vi "recon_zern_fileIO_MATLAB_v2.vi"(0 "Number of Phase":u32=2, 1 "Number for average":u32=2, 3 "Crop Size of image":u32=384, 4 "Background Value":u32=290, 5 "Zernike Order":u32=15, 7 "error in (no error)":errorcluster, 8 "Use GPU":bool=TRUE, 9 "Iteration Number":u32=10, 10 "idxType":enum16{"Wyant", "ANSI"}(ring), 12 "File Name":string="beads_1", 13 "Gamma Value":dbl=1e-06, 14 "Path In":path=path "D:/Data", 15 "Show Input":bool, 16 "Path Out":path=path "D:/Data", 17 "Show Recon":bool=TRUE) -> (20 "Zern coef out":sgl[](array[numeric]), 23 "Time cost (s)":dbl, 24 "RMSE Value":dbl, 27 "error out":errorcluster)   [LabVIEW 2018]
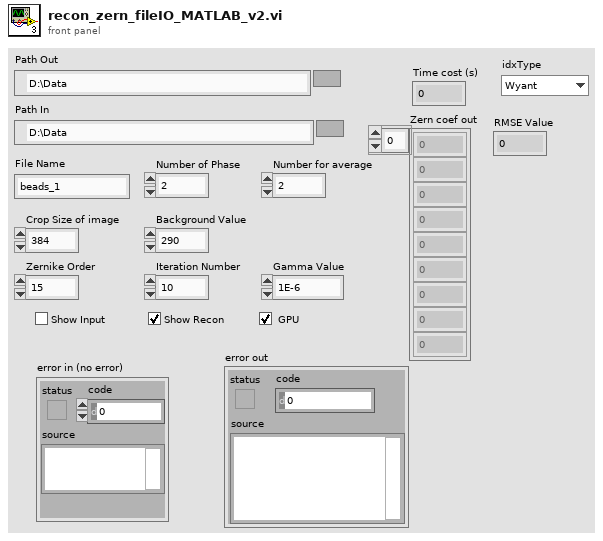
[diagram p1: front panel]
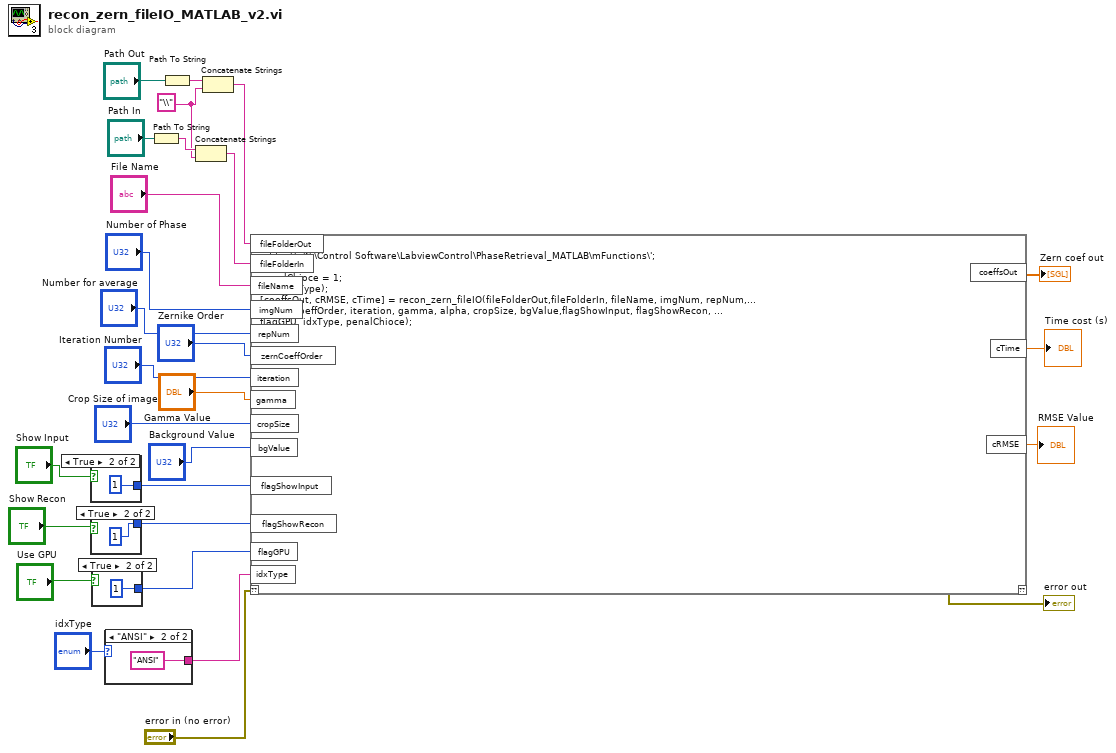
[diagram p0: block diagram]
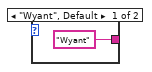
[diagram p2: hidden frame]
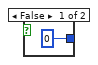
[diagram p3: hidden frame]
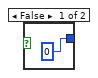
[diagram p4: hidden frame]
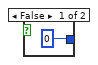
[diagram p5: hidden frame]
diagram:
  w7 = "\\"
  n1 = case shown="True" "Show Input" {
    tunnel: [0 1] -> w20
    frame False {
    }
    frame True {
    }
  }
  n2 = case shown="True" "Show Recon" {
    tunnel: [0 1] -> w19
    frame False {
    }
    frame True {
    }
  }
  n3 = case shown="True" "Use GPU" {
    tunnel: [0 1] -> w18
    frame False {
    }
    frame True {
    }
  }
  n4 = case shown="\"ANSI\"" "idxType" {
    tunnel: ["Wyant" "ANSI"] -> w1
    frame "Wyant", Default {
    }
    frame "ANSI" {
    }
  }
  n5 = Path To String(path="Path In") -> (string=w9:string)
  n6 = Path To String(path="Path Out") -> (string=w10:string)
  n7 = Concatenate Strings(w9, w7) -> (w6:string)
  n8 = Concatenate Strings(w10, w7) -> (w8:string)
  n9 = script code="close all;\naddpath 'C:\\Control Software\\LabviewControl\\PhaseRetrieval_MATLAB\\mFunctions\\';\nalpha = 0;\npenalChioce = 1;\ndisp(idxType);\n[coeffsOut, cRMSE, cTime] = recon_zern_fileIO(fileFolderOut,fileFolderIn, fileName, imgNum, repNum,...\n    zernCoeffOrder, iteration, gamma, alpha, cropSize, bgValue,flagShowInput, flagShowRecon, ...\nflagGPU, idxType, penalChioce);"("??"="error in (no error)", "fileFolderOut"=w8, "fileFolderIn"=w6, "fileName"="File Name", "imgNum"="Number of Phase", "repNum"="Number for average", "zernCoeffOrder"="Zernike Order", "iteration"="Iteration Number", "gamma"="Gamma Value", "cropSize"="Crop Size of image", "bgValue"="Background Value", "flagShowInput"=w20, "flagShowRecon"=w19, "flagGPU"=w18, "idxType"=w1) -> ("??"=→"error out":errorcluster, "coeffsOut"=→"Zern coef out":dbl[], "cTime"=→"Time cost (s)":dbl, "cRMSE"=→"RMSE Value":dbl)
